vi "Unbenannt 2.vi"() -> ()   [LabVIEW 2013]
panel:
  out "String":string
  in  "End Frequency (khz)":u32
  in  "Start Frequency (khz)":u32
  in  "Dwell Time (s)":dbl
  in  "Attenuation":u32
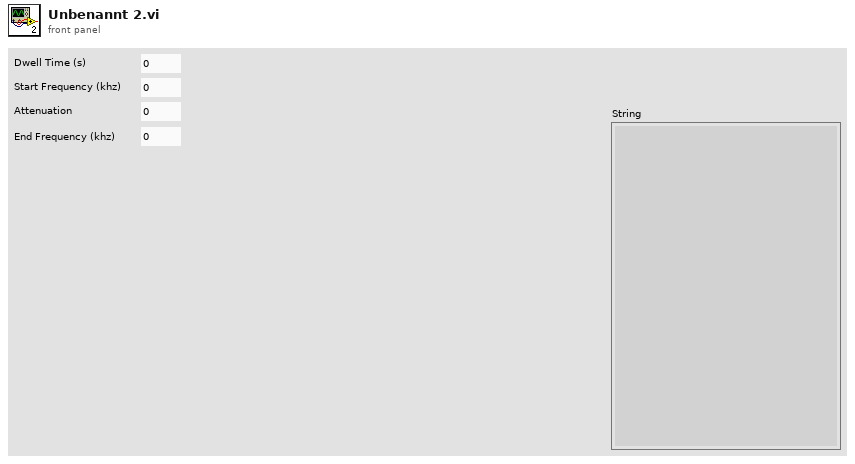
[diagram p1: front panel]
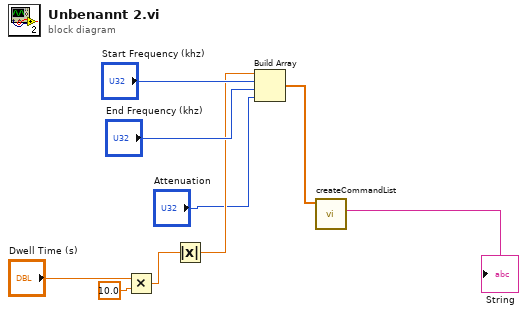
[diagram p0: block diagram]
diagram:
  n1 = Multiply(x="Dwell Time (s)", y=10.0) -> (x*y=w7:dbl)
  n2 = Absolute Value(x=w7) -> (abs(x)=w2:dbl)
  n3 = Build Array(w2, "Start Frequency (khz)", "End Frequency (khz)", "Attenuation") -> (w9:dbl[])
  n4 = call "createCommandList.vi"("Array"=w9) -> ("String"=→"String":string)  [unwired: 9 in]
